vi "MHL_file path updated.vi"(0 "Data Cluster in":T1, 1 "Settings":T6, 5 "error in (no error)":errorcluster, 8 "Message Queue in":refnum<class "Delacor_lib_QMH_Message Queue.lvclass">) -> (14 "Data Cluster out":T1, 19 "error out":errorcluster)   [LabVIEW 2019, in "Main UI.lvlib"]
uses:
  Main UI.lvlib
  Filepath Editor/Settings--cluster.ctl
  Module Data--cluster.ctl
  Class Library/XYgraph_class/XYgraph.lvclass
  FileReader/FPref_clustered--cluster references.ctl
  Main UI Shared/Boolean--FP cluster.ctl
  FileReader/FPref_cntrls--cluster references.ctl
  Main UI Shared/Indicators--FP cluster.ctl
  <vilib>/Delacor/Delacor QMH/Libraries/Message Queue_class/Delacor_lib_QMH_Message Queue.lvclass
  <vilib>/Utility/miscctls.llb/LVMinMaxIncTypeDef.ctl
  <vilib>/Delacor/Delacor QMH/Libraries/Message Queue_class/Delacor_lib_QMH_Message Queue.lvclass/Delacor_lib_QMH_Message Queue.ctl
  <vilib>/Delacor/Delacor QMH/Libraries/Message Queue_class/Delacor_lib_QMH_Enqueue Message (Single).vi
  Filepath Editor/Filepath Editor.lvlib
  Main UI Shared/MAIN UI Shared.lvlib
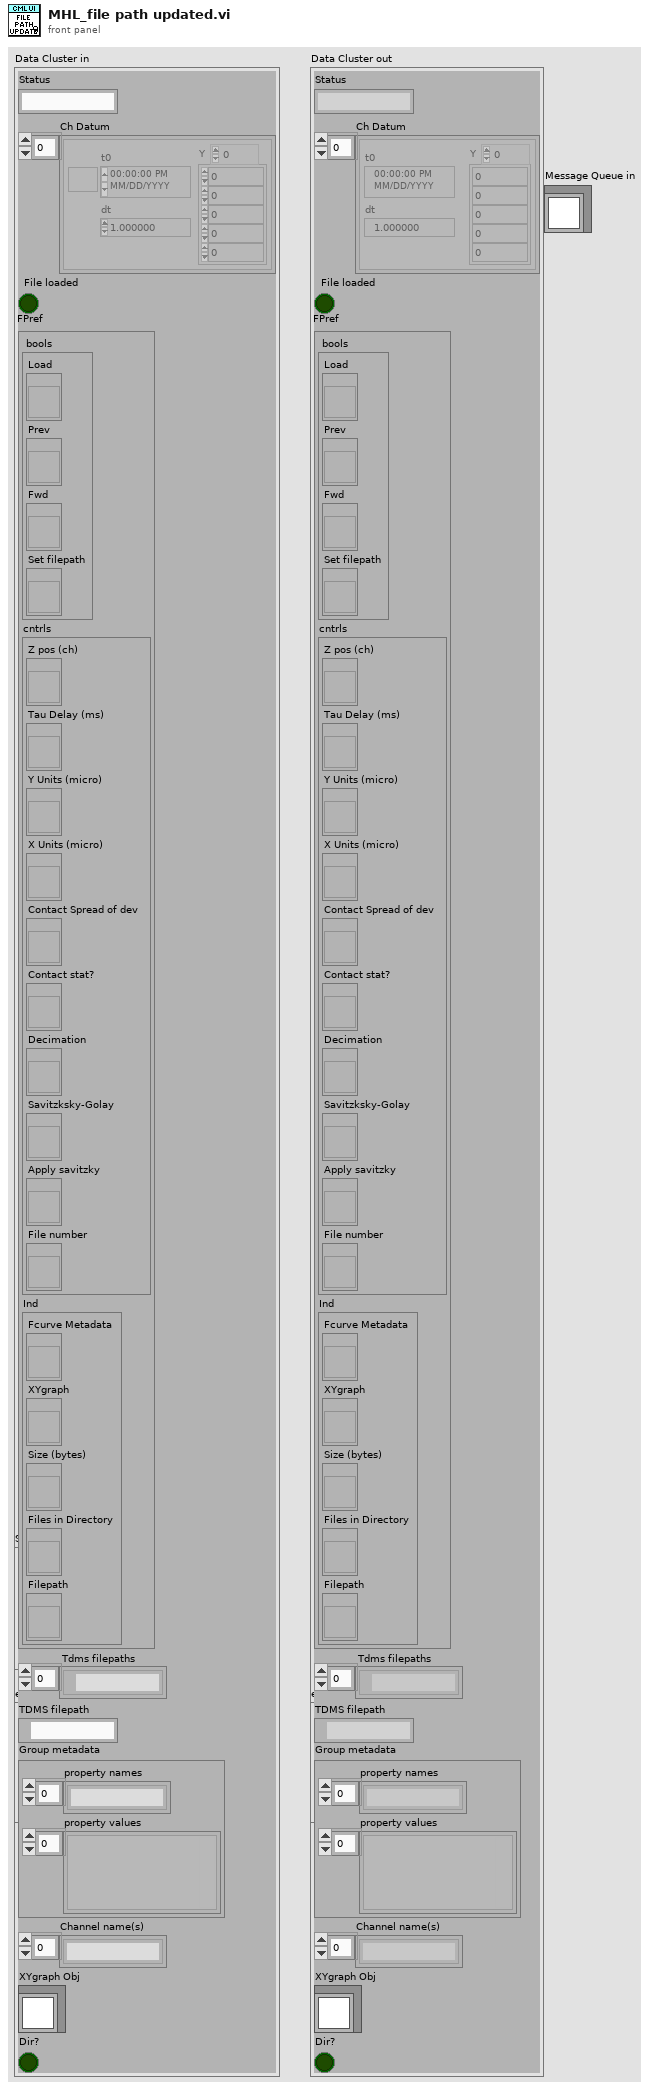
[diagram p1: front panel]
types:
  T1 = typedef "Main UI.lvlib/Module Data--cluster.ctl" = cluster{"Status":string, "Ch Datum":waveform(dbl)[], "File loaded":bool, "FPref":T2, "Tdms filepaths":path[], "TDMS filepath":path, "Group metadata":cluster{"property names":string[], "property values":variant[]}, "Channel name(s)":string[], "XYgraph Obj":refnum<class "XYgraph.lvclass">, "Dir?":bool}
  T2 = typedef "Main UI.lvlib/FPref_clustered--cluster references.ctl" = cluster{" bools":T3, "cntrls":T4, "Ind":T5}
  T3 = typedef "MAIN UI Shared.lvlib/Boolean--FP cluster.ctl" = cluster{"Load":refnum<vi>, "Prev":refnum<vi>, "Fwd":refnum<vi>, "Set filepath":refnum<vi>}
  T4 = typedef "Main UI.lvlib/FPref_cntrls--cluster references.ctl" = cluster{"Z pos (ch)":refnum<vi>, "Tau Delay (ms)":refnum<vi>, "Y Units (micro)":refnum<vi>, "X Units (micro)":refnum<vi>, "Contact Spread of dev":refnum<vi>, "Contact stat?":refnum<vi>, "Decimation":refnum<vi>, "Savitzksky-Golay":refnum<vi>, "Apply savitzky ":refnum<vi>, "File number":refnum<vi>}
  T5 = typedef "Main UI.lvlib/Indicators--FP cluster.ctl" = cluster{"Fcurve Metadata":refnum<vi>, "XYgraph":refnum<vi>, "Size (bytes)":refnum<vi>, "Files in Directory":refnum<vi>, "Filepath":refnum<vi>}
  T6 = typedef "Filepath Editor.lvlib/Settings--cluster.ctl" = cluster{"TDMS Filepath":path, "TDMS Directory":path, "Dir?":bool}
  T7 = typedef "LVMinMaxIncTypeDef.ctl" = cluster{"Minimum":dbl, "Maximum":dbl, "Increment":dbl}
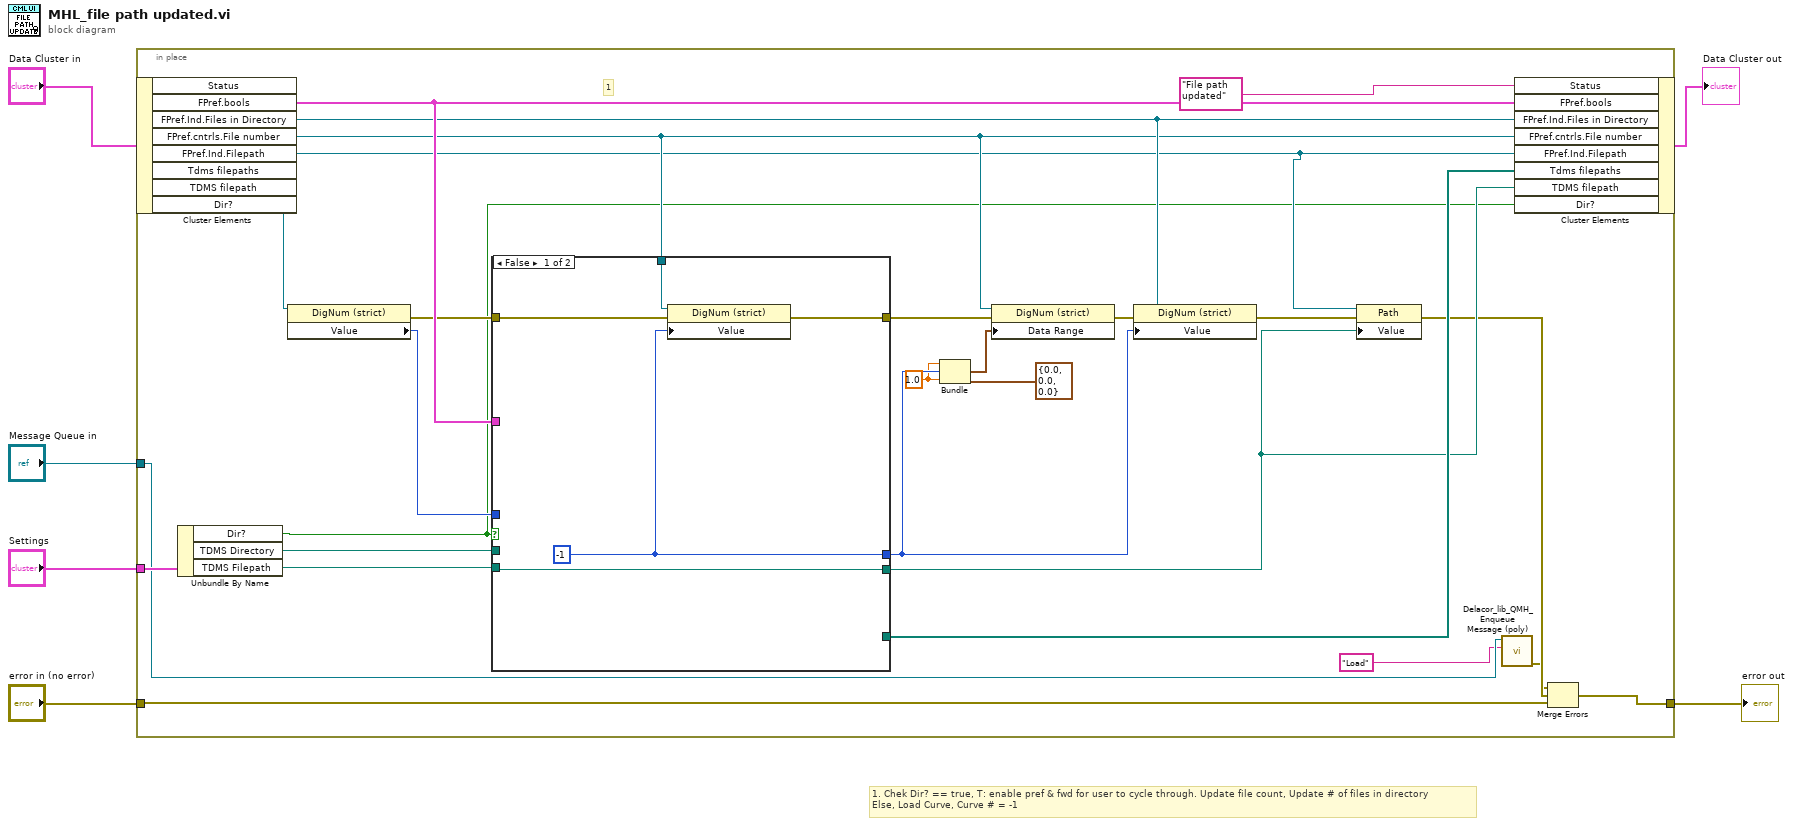
[diagram p0: block diagram]
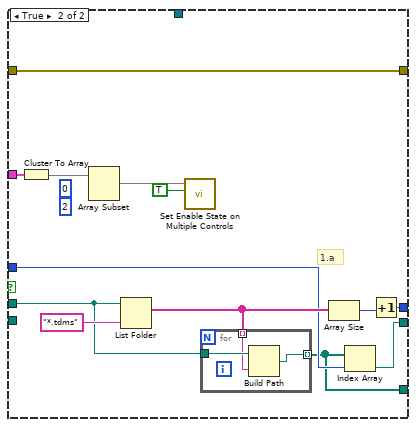
[diagram p2: hidden frame]
diagram:
  # "1. Chek Dir? == true, T: enable pref & fwd for user to cycle through. Update file count, Update # of files in directory\nElse, Load Curve, Curve # = -1"
  n1 = in-place {
    in-place-border: "Settings" -> [w31]
    in-place-border: "error in (no error)" -> [w30]
    in-place-border: [w29] -> w6
    in-place-border: "Message Queue in" -> [w9]
    w23 = 1.0 ("Increment")
    # "1"
    n2 = in-place-cluster #1("Data Cluster in") -> ("FPref.bools"=w28:T3, "FPref.Ind.Files in Directory"=w27:refnum<vi>, "FPref.cntrls.File number"=w20:refnum<vi>, "FPref.Ind.Filepath"=w19:refnum<vi>)  [unwired: 4 out]
    n3 = Unbundle By Name(w31) -> ("Dir?"=w7:bool, "TDMS Directory"=w18:path, "TDMS Filepath"=w22:path)
    n4 = property class="DigNum (strict)"(reference=w20) -> (error out=w12:errorcluster, "Value"=w21:i16)  [unwired: 1 in, 1 out]
    n5 = case shown="False" w7 {
      tunnel: w28 -> [_ w50]
      tunnel: [w36 w47] -> w24
      tunnel: w18 -> [_ w43]
      tunnel: w22 -> [w33 _]
      tunnel: w21 -> [_ w41]
      tunnel: w20 -> [w37 _]
      tunnel: [w33 w40] -> w16
      tunnel: [_ w39] -> w17
      tunnel: w12 -> [w34 w38]
      tunnel: [w35 w38] -> w11
      frame False {
        w36 = -1
        n6 = property class="DigNum (strict)"(reference=w37, error in=w34, "Value"=w36) -> (error out=w35:errorcluster)  [unwired: 1 out]
      }
      frame True {
        (unwired) 2 ("length")
        (unwired) 0 ("index")
        # "1.a"
        n7 = Cluster To Array(cluster=w50) -> (array=w46:refnum<vi>[])
        n8 = Array Subset(array=w46) -> (w45:refnum<vi>[])  [unwired: 2 in]
        n9 = List Folder(path=w43, pattern="*.tdms") -> (filenames=w42:string[])  [unwired: 2 in, 3 out]
        n10 = call "Set Enable State on Multiple Controls.vi"("Enable?"=TRUE, "Controls"=w45) -> ()  [unwired: 10 in]
        n11 = for {
          tunnel: w43 -> [w53]
          tunnel: w42 -> [w52] mode=indexing
          tunnel: [w51] -> w39 mode=indexing
          n12 = Build Path(base path=w53, name or relative path=w52) -> (appended path=w51:path)
        }
        n13 = Array Size(array=w42) -> (size(s)=w48:i32)
        n14 = Index Array(array=w39, index=w41) -> (element=w40:path)
        n15 = Increment(x=w48) -> (x+1=w47:i32)
      }
    }
    n16 = Bundle(cluster=T7 {"Minimum"=0.0, "Maximum"=0.0, "Increment"=0.0} ("Data Entry Limits"), "Minimum"=w23, "Maximum"=w24, "Increment"=w23) -> (w25:T7)
    n17 = property class="DigNum (strict)"(reference=w20, error in=w11, "Data Range"=w25) -> (error out=w15:errorcluster)  [unwired: 1 out]
    n18 = property class="DigNum (strict)"(reference=w27, error in=w15, "Value"=w24) -> (error out=w14:errorcluster)  [unwired: 1 out]
    n19 = property class="Path"(reference=w19, error in=w14, "Value"=w16) -> (error out=w13:errorcluster)  [unwired: 1 out]
    n20 = call-poly <vilib>:"Delacor_lib_QMH_Enqueue Message (poly).vi"("Message"="Load", "Message Queue in"=w9) -> ("error out"=w10:errorcluster)  [unwired: 8 in, 1 out]
    n21 = in-place-cluster #1("Status"="File path updated", "FPref.bools"=w28, "FPref.Ind.Files in Directory"=w27, "FPref.cntrls.File number"=w20, "FPref.Ind.Filepath"=w19, "Tdms filepaths"=w17, "TDMS filepath"=w16, "Dir?"=w7) -> (→"Data Cluster out":T1)
    n22 = Merge Errors(w10, w13, w30) -> (w29:errorcluster)
  }
  "error out" <- w6
